vi "CleanReplies.vi"(11 "help in":string) -> (2 "body":string, 3 "header":string)   [LabVIEW 2021]
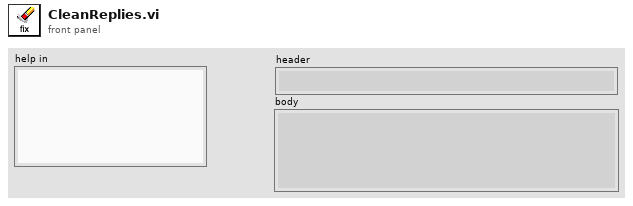
[diagram p1: front panel]
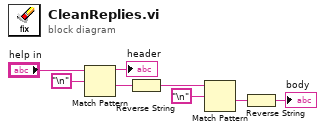
[diagram p0: block diagram]
diagram:
  n1 = Match Pattern(string="help in", regular expression="\n") -> (before substring=→"header":string, after substring=w2:string)  [unwired: 1 in, 2 out]
  n2 = Reverse String(1:w2) -> (0:w3:string)
  n3 = Match Pattern(string=w3, regular expression="\n") -> (after substring=w5:string)  [unwired: 1 in, 3 out]
  n4 = Reverse String(1:w5) -> (0:→"body":string)
